vi "SCLN_CheckOldAuthentication.vi"(0 "Server Name":string, 1 "TCP IN":refnum<k5>) -> (2 "TCP OUT":refnum<k5>, 3 "Client Index":i32, 4 "Authentic":bool, 5 "error out":errorcluster)   [LabVIEW 2015]
panel:
  in  "error out":errorcluster
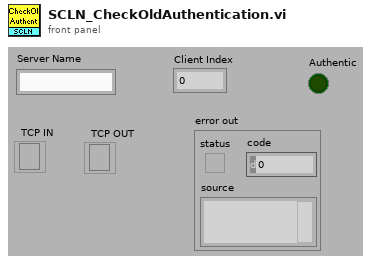
[diagram p1: front panel]
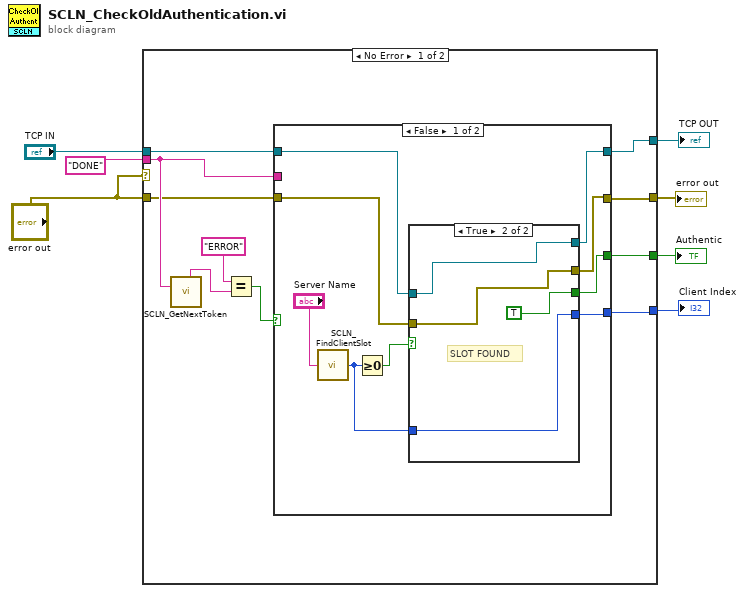
[diagram p0: block diagram]
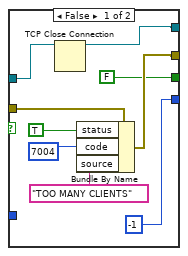
[diagram p2: hidden frame]
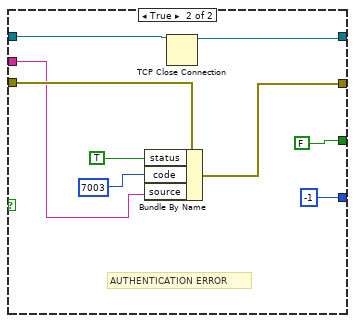
[diagram p3: hidden frame]
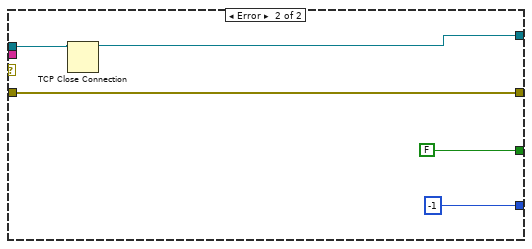
[diagram p4: hidden frame]
diagram:
  n1 = case shown="No Error" "error out" {
    tunnel: "TCP IN" -> [w14 w53]
    tunnel: "DONE" -> [w13 _]
    tunnel: "error out" -> [w9 w52]
    tunnel: [w8 w52] -> w2
    tunnel: [w11 FALSE] -> w7
    tunnel: [w10 -1] -> w6
    tunnel: [w12 w49] -> w5
    frame No Error {
      n2 = call "SCLN_GetNextToken.vi"("Input string"=w13) -> ("Token"=w17:string)  [unwired: 4 in, 1 out]
      n3 = Equal?(x="ERROR", y=w17) -> (x = y?=w15:bool)
      n4 = case shown="False" w15 {
        tunnel: w14 -> [w22 w41]
        tunnel: w13 -> [_ w43]
        tunnel: [w18 w40] -> w12
        tunnel: [w20 FALSE] -> w11
        tunnel: [w21 -1] -> w10
        tunnel: w9 -> [w23 w46]
        tunnel: [w19 w42] -> w8
        frame False {
          n5 = call "SCLN_FindClientSlot.vi"("Server Name"="Server Name") -> ("Client Index"=w24:i32)
          n6 = Greater Or Equal To 0?(x=w24) -> (x >= 0?=w25:bool)
          n7 = case shown="True" w25 {
            tunnel: w24 -> [_ w39]
            tunnel: w23 -> [w35 w37]
            tunnel: w22 -> [w31 w36]
            tunnel: [-1 w39] -> w21
            tunnel: [FALSE TRUE] -> w20
            tunnel: [w29 w37] -> w19
            tunnel: [w30 w36] -> w18
            frame False {
              n8 = TCP Close Connection(connection ID=w31) -> (connection ID out=w30:refnum<k5>)  [unwired: 2 in, 1 out]
              n9 = Bundle By Name(cluster=w35, "status"=TRUE, "code"=7004, "source"="TOO MANY CLIENTS") -> (w29:errorcluster)
            }
            frame True {
              # "SLOT FOUND"
            }
          }
        }
        frame True {
          # "AUTHENTICATION ERROR"
          n10 = Bundle By Name(cluster=w46, "status"=TRUE, "code"=7003, "source"=w43) -> (w42:errorcluster)
          n11 = TCP Close Connection(connection ID=w41) -> (connection ID out=w40:refnum<k5>)  [unwired: 2 in, 1 out]
        }
      }
    }
    frame Error {
      n12 = TCP Close Connection(connection ID=w53) -> (connection ID out=w49:refnum<k5>)  [unwired: 2 in, 1 out]
    }
  }
  "Client Index" <- w6
  "Authentic" <- w7
  "TCP OUT" <- w5
  "error out" <- w2
